vi "Boolean String to Boolean.vi"(1 "T/F String":string) -> (0 "Value":bool)   [LabVIEW 2012, in "CS++Base.lvlib"]
doc: "Convert Boolean string to boolean."
uses:
  CS++Base.lvlib
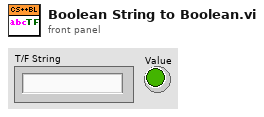
[diagram p1: front panel]
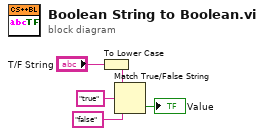
[diagram p0: block diagram]
diagram:
  n1 = To Lower Case(string="T/F String") -> (all lower case string=w5:string)
  n2 = Match True/False String(2:"false" ("string"), 3:"true" ("true string"), 4:w5) -> (0:→"Value":bool)  [unwired: 1 out]
